vi "Ex_Lookup TDMSupport.vi"(8 "error in (no error)":errorcluster, 11 "VI RefNum for Context":refnum<vi>) -> (0 "error out":errorcluster, 1 "TDMS Support":bool, 2 "TDM Support?":bool, 3 "VI RefNum Out":refnum<vi>)   [LabVIEW 2017]
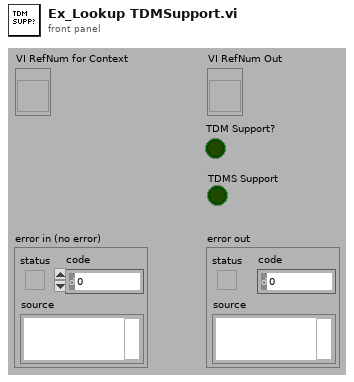
[diagram p1: front panel]
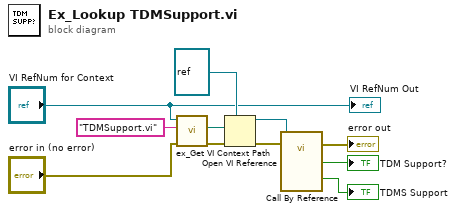
[diagram p0: block diagram]
diagram:
  n1 = call <vilib>:"ex_Get VI Context Path.vi"("error in (no error)"="error in (no error)", "File Name"="TDMSupport.vi", "VI RefNum for Context"="VI RefNum for Context") -> ("error out"=w5:errorcluster, "Resulting File Path"=w8:path)  [unwired: 7 in]
  n2 = Open VI Reference(type specifier VI Refnum (for type only)=refnum<vi> refnum ("reference"), vi path=w8, error in (no error)=w5) -> (vi reference=w10:refnum<vi>, error out=w9:errorcluster)  [unwired: 3 in]
  n3 = call-by-ref "?"(reference=w10, error in=w9) -> (error out=→"error out":errorcluster, "TDMS Support"=→"TDMS Support":bool, "TDM Support"=→"TDM Support?":bool)  [unwired: 2 in, 1 out]
  "VI RefNum Out" <- "VI RefNum for Context"
